vi "Out_S7F17.vi"(8 "error in (no error)":errorcluster, 10 "PPID":string[](array[string]), 11 "S7 Message Class in":refnum<class "S7 Message Class.lvclass">) -> (0 "error out":errorcluster, 3 "S7 Message Class out":refnum<class "S7 Message Class.lvclass">)   [LabVIEW 2020, in "SECS Communication.lvlib" / "S7 Message Class.lvclass"]
uses:
  S7 Message Class.lvclass
  D:/Dropbox/SECS/LabVIEW Code/Com/SECS Communication/SECS-II Class/SECS-II Class.lvclass
  SECS-II Class/Data Message_List.vi
  SECS-II Class/Data Message_ASCII.vi
  S7 Message Class.lvclass/S7 Message Class.ctl
  SECS-II Class/SECS-II Class.lvclass
  D:/Dropbox/SECS/LabVIEW Code/Com/SECS Communication/S7 Message Class/S7 Message Class.lvclass
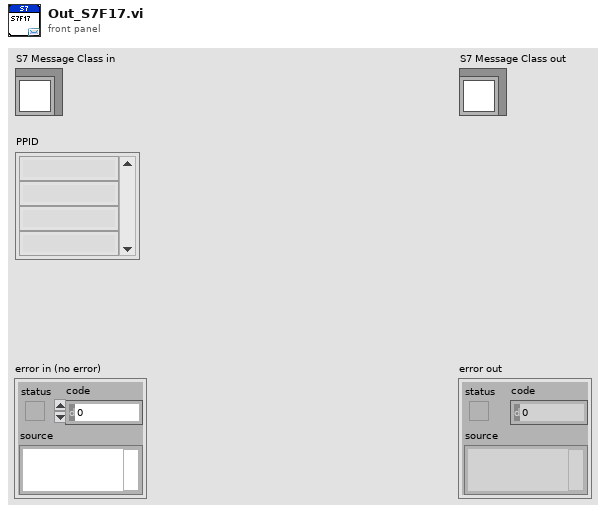
[diagram p1: front panel]
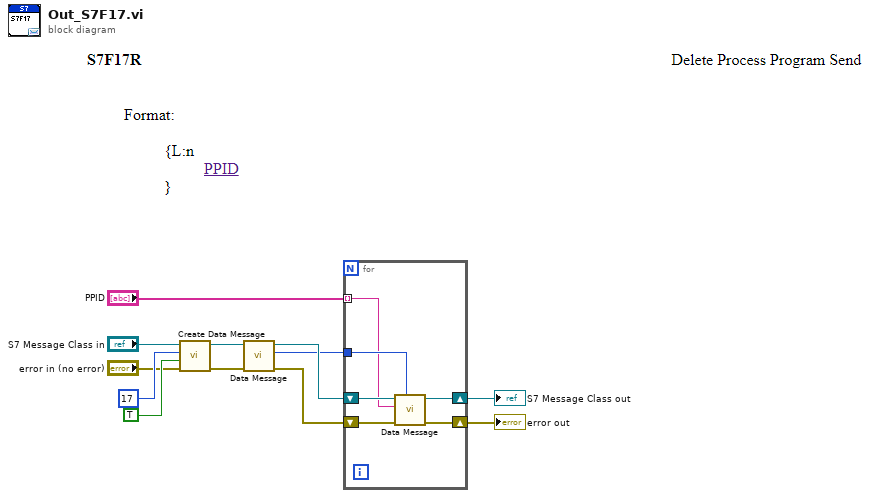
[diagram p0: block diagram]
diagram:
  n1 = call "Create Data Message.vi"("error in (no error)"="error in (no error)", "W-Bit"=TRUE, "Function"=u8 17, "SECS-II Class in"="S7 Message Class in") -> ("error out"=w4:errorcluster, "SECS-II Class out"=w5:refnum<class "S7 Message Class.lvclass">)  [unwired: 6 in]
  n2 = call-poly "Data Message.vi"("error in"=w4, "SECS-II Class in"=w5) -> ("error out"=w7:errorcluster, "Index"=w6:i32, "SECS-II Class out"=w8:refnum<class "S7 Message Class.lvclass">)  [unwired: 7 in]
  n3 = for {
    tunnel: w6 -> [w16]
    shift-right: [w15] -> w2
    shift-left: w8 -> [w18]
    shift-right: [w14] -> w1
    shift-left: w7 -> [w17]
    tunnel: "PPID" -> [w13] mode=indexing
    n4 = call-poly "Data Message.vi"("Parent Index"=w16, "error in"=w17, "Data"=w13, "SECS-II Class in"=w18) -> ("error out"=w14:errorcluster, "SECS-II Class out"=w15:refnum<class "S7 Message Class.lvclass">)  [unwired: 6 in]
  }
  "error out" <- w1
  "S7 Message Class out" <- w2
